vi "save_xml.vi"(8 "error in":errorcluster, 10 "base path":path, 11 "DAQmx Pulse Settings":T1={"Enable DAQmx Pulses"=FALSE, "DAQmx Physical Channels"="Dev2/port0_32", "Clock Rate"=10000000.0, "units per second"=1000.0, "Start Trigger"={"Wait for start trigger?"=FALSE, "source"="/Dev1/PFI0", "edge"=10280}, "Timing Sequence Control (ms)"=[["camera/repump", "1", "0", "", "", "", "", "", "", "", "", "", "", "", "", "", "", "", "", "", "1000", "1000", "1000", "1000", "", "", "", "", "", "", "", "", "", "", "", "", "", "", ""], ["probe", "1", "0", "", "", "", "", "", "", "", "", "", "", "", "", "", "", "", "", "", "", "", "", "", "", "", "", "", "", "", "", "", "", "", "", "", "", "", ""], ["bias field", "1", "0", "", "", "", "", "", "", "", "", "", "", "", "", "", "", "", "", "", "", "", "", "", "", "", "", "", "", "", "", "", "", "", "", "", "", "", ""], ["switch 1 MOT to PGC freq shift", "1", "0", "", "", "", "", "", "", "", "", "", "", "", "", "", "", "", "", "", "", "", "", "", "", "", "", "", "", "", "", "", "", "", "", "", "", "", ""], ["B field", "1", "0", "", "", "", "", "", "", "", "", "", "", "", "", "", "", "", "", "", "", "", "", "", "", "", "", "", "", "", "", "", "", "", "", "", "", "", ""], ["trigger PD1", "1", "0", "", "", "", "", "", "", "", "", "", "", "", "", "", "", "", "", "", "", "", "", "", "", "", "", "", "", "", "", "", "", "", "", "", "", "", ""], ["rf switch 2 cooling laser on/off", "1", "0", "", "", "", "", "", "", "", "", "", "", "", "", "", "", "", "", "", "", "", "", "", "", "", "", "", "", "", "", "", "", "", "", "", "", "", ""], ["Bob switch", "1", "0", "", "", "", "", "", "", "", "", "", "", "", "", "", "", "", "", "", "", "", "", "", "", "", "", "", "", "", "", "", "", "", "", "", "", "", ""], ["switch 3 894nm", "1", "0", "", "", "", "", "", "", "", "", "", "", "", "", "", "", "", "", "", "", "", "", "", "", "", "", "", "", "", "", "", "", "", "", "", "", "", ""], ["clock trigger", "1", "0", "", "", "", "", "", "", "", "", "", "", "", "", "", "", "", "", "", "", "", "", "", "", "", "", "", "", "", "", "", "", "", "", "", "", "", ""], ["Raman", "1", "0", "", "", "", "", "", "", "", "", "", "", "", "", "", "", "", "", "", "", "", "", "", "", "", "", "", "", "", "", "", "", "", "", "", "", "", ""], ["684 shutter", "1", "0", "", "", "", "", "", "", "", "", "", "", "", "", "", "", "", "", "", "", "", "", "", "", "", "", "", "", "", "", "", "", "", "", "", "", "", ""], ["repumper switch 2", "1", "0", "", "", "", "", "", "", "", "", "", "", "", "", "", "", "", "", "", "", "", "", "", "", "", "", "", "", "", "", "", "", "", "", "", "", "", ""], ["further PGC", "1", "0", "", "", "", "", "", "", "", "", "", "", "", "", "", "", "", "", "", "", "", "", "", "", "", "", "", "", "", "", "", "", "", "", "", "", "", ""], ["pumping laser switch 2", "1", "0", "", "", "", "", "", "", "", "", "", "", "", "", "", "", "", "", "", "", "", "", "", "", "", "", "", "", "", "", "", "", "", "", "", "", "", ""], ["Raman 2", "1", "0", "", "", "", "", "", "", "", "", "", "", "", "", "", "", "", "", "", "", "", "", "", "", "", "", "", "", "", "", "", "", "", "", "", "", "", ""], ["MOT beam on/off switch 2", "1", "0", "", "", "", "", "", "", "", "", "", "", "", "", "", "", "", "", "", "", "", "", "", "", "", "", "", "", "", "", "", "", "", "", "", "", "", ""], ["push beam switch 2", "1", "0", "", "", "", "", "", "", "", "", "", "", "", "", "", "", "", "", "", "", "", "", "", "", "", "", "", "", "", "", "", "", "", "", "", "", "", ""], ["532 AOM", "1", "0", "", "", "", "", "", "", "", "", "", "", "", "", "", "", "", "", "", "", "", "", "", "", "", "", "", "", "", "", "", "", "", "", "", "", "", ""], ["Andor Luca Trigger", "1", "0", "", "", "", "", "", "", "", "", "", "", "", "", "", "", "", "", "", "", "", "", "", "", "", "", "", "", "", "", "", "", "", "", "", "", "", ""], ["trigger PD2", "1", "0", "", "", "", "", "", "", "", "", "", "", "", "", "", "", "", "", "", "", "", "", "", "", "", "", "", "", "", "", "", "", "", "", "", "", "", ""], ["1038 switch", "1", "0", "", "", "", "", "", "", "", "", "", "", "", "", "", "", "", "", "", "", "", "", "", "", "", "", "", "", "", "", "", "", "", "", "", "", "", ""], ["459 switch", "1", "0", "", "", "", "", "", "", "", "", "", "", "", "", "", "", "", "", "", "", "", "", "", "", "", "", "", "", "", "", "", "", "", "", "", "", "", ""], ["", "", "", "", "", "", "", "", "", "", "", "", "", "", "", "", "", "", "", "", "", "", "", "", "", "", "", "", "", "", "", "", "", "", "", "", "", "", ""], ["", "", "", "", "", "", "", "", "", "", "", "", "", "", "", "", "", "", "", "", "", "", "", "", "", "", "", "", "", "", "", "", "", "", "", "", "", "", ""], ["", "", "", "", "", "", "", "", "", "", "", "", "", "", "", "", "", "", "", "", "", "", "", "", "", "", "", "", "", "", "", "", "", "", "", "", "", "", ""], ["", "", "", "", "", "", "", "", "", "", "", "", "", "", "", "", "", "", "", "", "", "", "", "", "", "", "", "", "", "", "", "", "", "", "", "", "", "", ""], ["", "", "", "", "", "", "", "", "", "", "", "", "", "", "", "", "", "", "", "", "", "", "", "", "", "", "", "", "", "", "", "", "", "", "", "", "", "", ""], ["", "", "", "", "", "", "", "", "", "", "", "", "", "", "", "", "", "", "", "", "", "", "", "", "", "", "", "", "", "", "", "", "", "", "", "", "", "", ""], ["", "", "", "", "", "", "", "", "", "", "", "", "", "", "", "", "", "", "", "", "", "", "", "", "", "", "", "", "", "", "", "", "", "", "", "", "", "", ""], ["", "", "", "", "", "", "", "", "", "", "", "", "", "", "", "", "", "", "", "", "", "", "", "", "", "", "", "", "", "", "", "", "", "", "", "", "", "", ""], ["", "", "", "", "", "", "", "", "", "", "", "", "", "", "", "", "", "", "", "", "0", "", "", "", "", "", "", "", "", "", "", "", "", "", "", "", "", "", ""]]} {"Start Trigger"."edge" items=["Rising"=10280, "Falling"=10171]; "Clock Rate" min=0.0 max=200000000.0 format="%.2p"}) -> (0 "error out":errorcluster)   [LabVIEW 2012, in "DAQmx_pulse_out.lvclass"]
uses:
  DAQmx_pulse_out.lvclass
  settings.ctl
  <vilib>/Utility/xml.llb/Write to XML File(string).vi
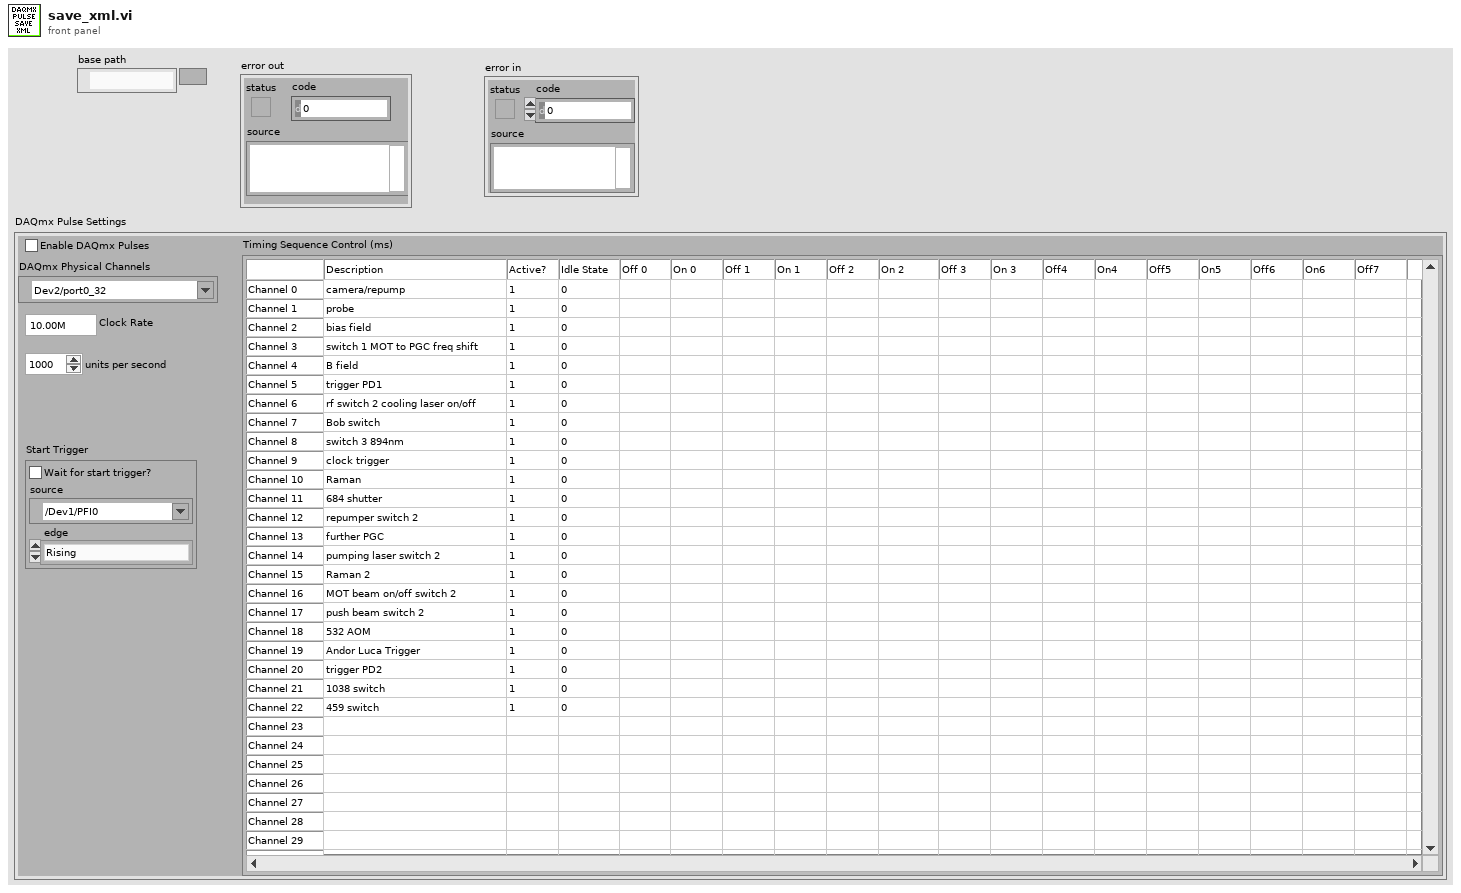
[diagram p1: front panel]
types:
  T1 = typedef "DAQmx_pulse_out.lvclass/settings.ctl" = cluster{"Enable DAQmx Pulses":bool, "DAQmx Physical Channels":tag, "Clock Rate":dbl, "units per second":dbl, "Start Trigger":cluster{"Wait for start trigger?":bool, "source":tag, "edge":i32}, "Timing Sequence Control (ms)":string[][]}
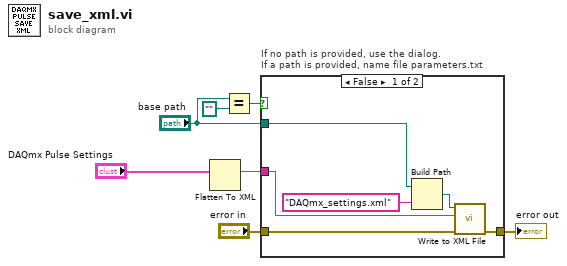
[diagram p0: block diagram]
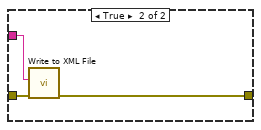
[diagram p2: hidden frame]
diagram:
  n1 = Flatten To XML(anything="DAQmx Pulse Settings") -> (xml string=w2:string)
  n2 = Equal?(x="base path", y=path "") -> (x = y?=w5:bool)
  n3 = case "If no path is provided, use the dialog.\nIf a path is provided, name file parameters.txt" shown="False" w5 {
    tunnel: [w9 w15] -> w6
    tunnel: "base path" -> [w12 _]
    tunnel: "error in" -> [w10 w16]
    tunnel: w2 -> [w8 w14]
    frame False {
      n4 = Build Path(base path=w12, name or relative path="DAQmx_settings.xml") -> (appended path=w11:path)
      n5 = call-poly <vilib>:"Write to XML File.vi"("error in (no error)"=w10, "XML Input"=w8, "XML File Path"=w11) -> ("error out"=w9:errorcluster)  [unwired: 6 in, 2 out]
    }
    frame True {
      n6 = call-poly <vilib>:"Write to XML File.vi"("error in (no error)"=w16, "XML Input"=w14) -> ("error out"=w15:errorcluster)  [unwired: 7 in, 2 out]
    }
  }
  "error out" <- w6
